vi "Archon RAW to FITS MAIN.vi"() -> ()   [LabVIEW 2023]
uses:
  gfitsio.lvlib
  cfitsio-bitpix.ctl
  gfitsio-write-image-subset-i16-2d.vi
  <vilib>/picture/picture.llb/Draw True-Color Pixmap.vi
  gfitsio-read-image-subset-i32-2d.vi
panel:
  out "hdu names":string[](array[string])=["Primary", "test3.fits"]
  out "hdu name":string="test3.fits"
  in  "Tab Control":enum32{"Complete Image", "Red", "Green", "Blue"}(tab)
  out "Complete Image":picture
  out "Red":picture
  out "Green":picture
  out "Blue":picture
  in  "save binary":path=path "D:/OCI Backups/600__2018_03_12-12.51.07.bin"
  out "Image Data":u16[][](graph)
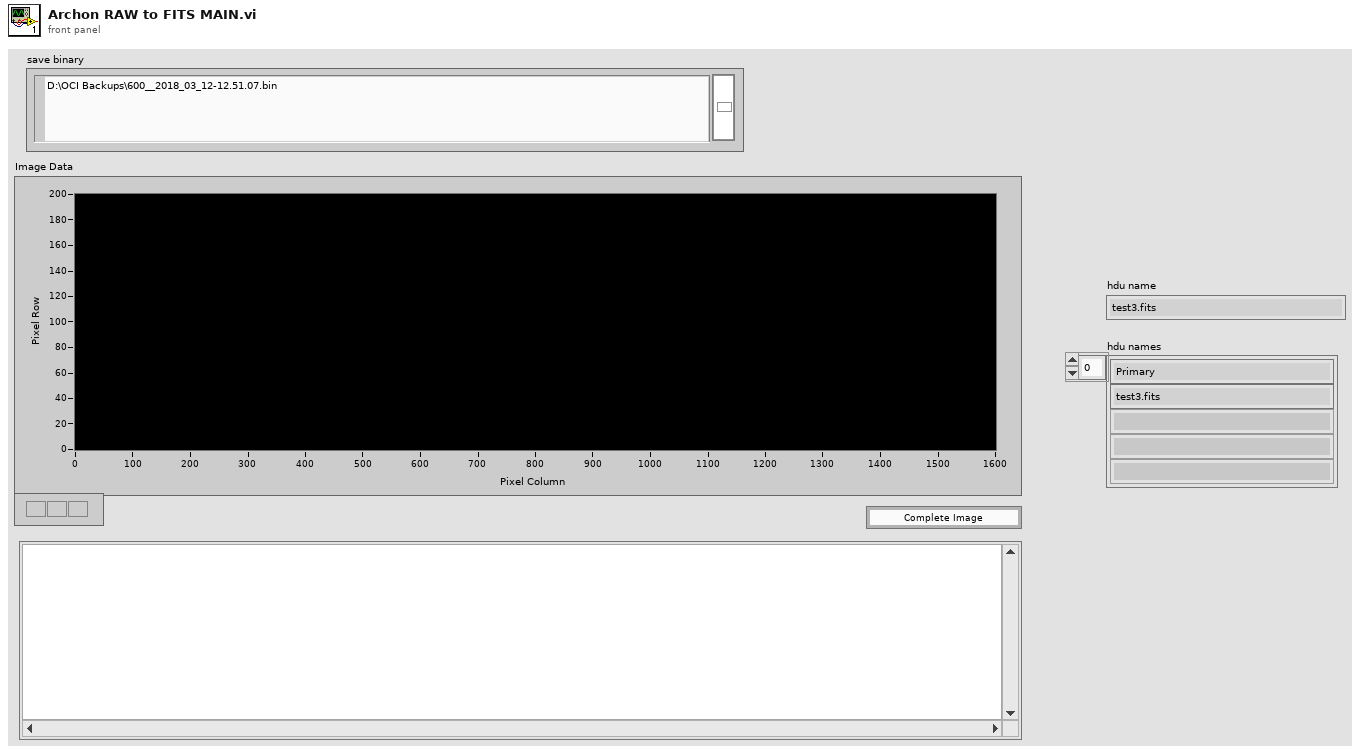
[diagram p1: front panel]
types:
  T1 = enum16{"big-endian, network order", "native, host order", "little-endian"}
  T2 = enum16{"open", "replace", "create", "open or create", "replace or create", "replace or create with confirmation"}
  T3 = enum16{"open", "open or create", "create", "create or replace"}
  T4 = enum16{"open", "open or create", "create or replace", "create", "open (read only)"}
  T5 = typedef "gfitsio.lvlib/cfitsio-bitpix.ctl" = i32
  T6 = typedef "gfitsio.lvlib/gfitsio-refnum.ctl" = refnum<k1>
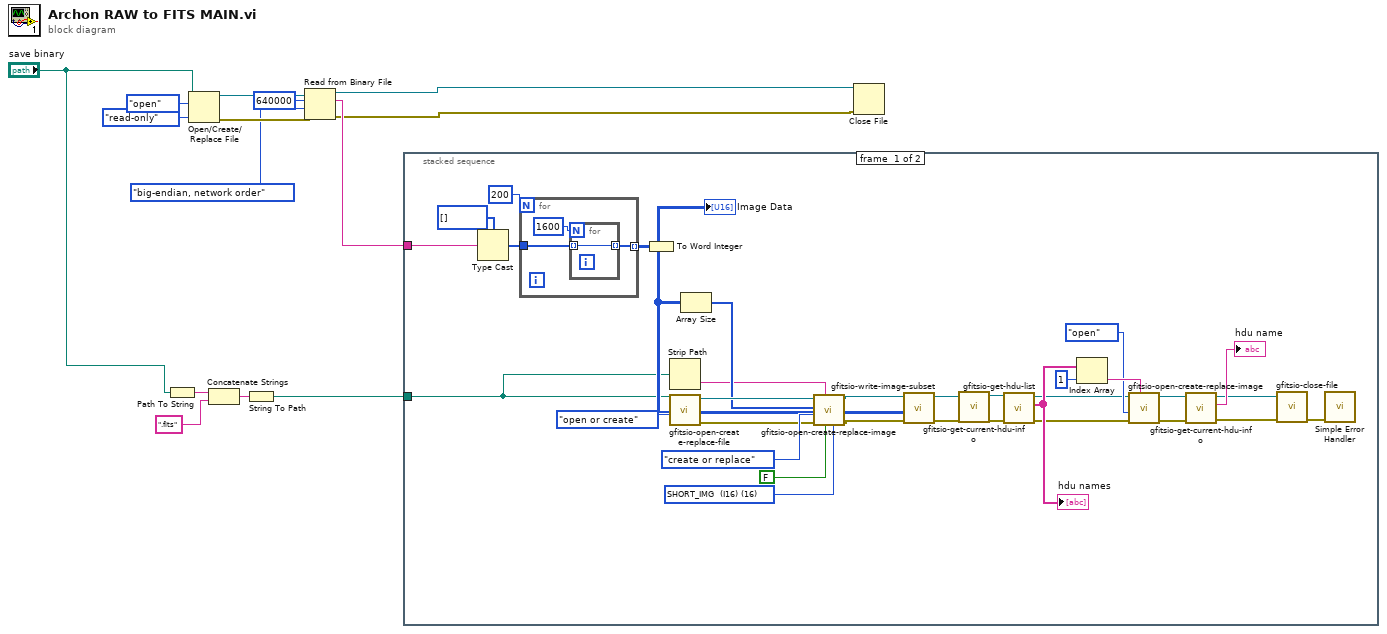
[diagram p0: block diagram]
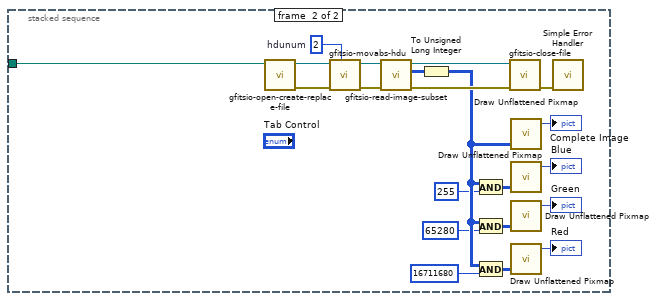
[diagram p2: hidden frame]
diagram:
  n1 = Path To String(path="save binary") -> (string=w5:string)
  n2 = Open/Create/Replace File(file path (use dialog)="save binary", operation (0:open)=T2."open", access (0:read/write)=enum16{"read/write", "read-only", "write-only"}."read-only") -> (refnum out=w12:refnum<file>, error out=w11:errorcluster)  [unwired: 3 in, 1 out]
  n3 = Concatenate Strings(w5, ".fits" ("string")) -> (w3:string)
  n4 = String To Path(string=w3) -> (path=w1:path)
  n5 = Read from Binary File(8:w11, 9:T1."big-endian, network order" ("byte order (0:big-endian, network order)"), 10:640000 ("count (1)"), 11:w12) -> (0:w6:errorcluster, 2:w8:string, 3:w7:refnum<file>)  [unwired: 2 in, 1 out]
  n6 = stacked-sequence {
    tunnel: w8 -> [w45 _]
    tunnel: w1 -> [w15 w51]
    frame #0 {
      w41 = T5 16 items=["<invalid type>"=0, "BYTE_IMG  (U8)"=8, "SHORT_IMG  (I16)"=16, "USHORT_IMG  (U16)"=20, "LONG_IMG  (I32)"=32, "ULONG_IMG  (U32)"=40, "FLOAT_IMG  (SGL)"=-32, "DOUBLE_IMG  (DBL)"=-64] ("image data type")
      n7 = Type Cast(type=u16[] [], x=w45) -> (*(type *) &x=w44:u16[])
      n8 = for {
        N: 200 ("dimension size") -> [_]
        tunnel: w44 -> [w49]
        tunnel: [w48] -> w18 mode=indexing
        n9 = for {
          N: 1600 ("dimension size") -> [_]
          tunnel: w49 -> [w50] mode=indexing
          tunnel: [w50] -> w48 mode=indexing
        }
      }
      "Image Data" <- w18
      n10 = To Word Integer(number=w18) -> ()  [unwired: 1 out]
      n11 = Strip Path(path=w15) -> (name=w16:string)  [unwired: 1 out]
      n12 = call "gfitsio-open-create-replace-file.vi"("function (open)"=T4."open or create", "file path (dialog if empty)"=w15) -> ("error out"=w38:errorcluster, "gfits refnum"=w37:T6)  [unwired: 7 in, 1 out]
      n13 = Array Size(array=w18) -> (size(s)=w36:i32[])
      n14 = call "gfitsio-open-create-replace-image.vi"("image data type"=w41, "advisory dialog? (display:T)"=FALSE, "hdu name (dialog if empty)"=w16, "error in (no error)"=w38, "function (create or replace)"=T3."create or replace" ("function (open or create)"), "naxes"=w36, "gfits refnum"=w37) -> ("error out"=w19:errorcluster, "dup gfits refnum"=w20:T6)  [unwired: 2 in, 1 out]
      n15 = call-poly "gfitsio-write-image-subset.vi"("error in (no error)"=w19, "data"=w18, "gfits refnum"=w20) -> ("error out"=w23:errorcluster, "dup gfits refnum"=w22:T6)  [unwired: 7 in]
      n16 = call "gfitsio-get-current-hdu-info.vi"("error in (no error)"=w23, "gfits refnum"=w22) -> ("error out"=w25:errorcluster, "dup gfits refnum"=w24:T6)  [unwired: 5 in, 3 out]
      n17 = call "gfitsio-get-hdu-list.vi"("error in (no error)"=w25, "gfits refnum"=w24) -> ("error out"=w27:errorcluster, "hdu names"=w33:string[], "dup gfits refnum"=w26:T6)  [unwired: 6 in, 1 out]
      "hdu names" <- w33
      n18 = Index Array(array=w33, index=1) -> (element=w34:string)
      n19 = call "gfitsio-open-create-replace-image.vi"("hdu name (dialog if empty)"=w34, "error in (no error)"=w27, "function (create or replace)"=T3."open", "gfits refnum"=w26) -> ("error out"=w30:errorcluster, "dup gfits refnum"=w29:T6)  [unwired: 5 in, 1 out]
      n20 = call "gfitsio-get-current-hdu-info.vi"("error in (no error)"=w30, "gfits refnum"=w29) -> ("error out"=w31:errorcluster, "hdu name"=→"hdu name":string, "dup gfits refnum"=w17:T6)  [unwired: 5 in, 2 out]
      n21 = call "gfitsio-close-file.vi"("error in (no error)"=w31, "gfits refnum"=w17) -> ("error out"=w21:errorcluster)  [unwired: 8 in, 1 out]
      n22 = call <vilib>:"Simple Error Handler.vi"("error in (no error)"=w21) -> ()  [unwired: 4 in, 5 out]
    }
    frame #1 {
      w52 = 2  # hdunum
      n23 = call "gfitsio-open-create-replace-file.vi"("file path (dialog if empty)"=w51) -> ("error out"=w71:errorcluster, "gfits refnum"=w70:T6)  [unwired: 8 in, 1 out]
      n24 = call "gfitsio-movabs-hdu.vi"("hdunum"=w52, "error in (no error)"=w71, "gfits refnum"=w70) -> ("error out"=w69:errorcluster, "dup gfits refnum"=w68:T6)  [unwired: 6 in, 1 out]
      n25 = call-poly "gfitsio-read-image-subset.vi"("error in (no error)"=w69, "gfits refnum"=w68) -> ("error out"=w67:errorcluster, "data"=w64:i32[][], "dup gfits refnum"=w66:T6)  [unwired: 7 in]
      n26 = To Unsigned Long Integer(number=w64) -> (unsigned 32bit integer=w56:u32[][])
      n27 = And(x=w56, y=u32 255) -> (x .and. y?=w63:u32[][])
      n28 = And(x=w56, y=u32 65280) -> (x .and. y?=w60:u32[][])
      n29 = And(x=w56, y=u32 16711680) -> (x .and. y?=w58:u32[][])
      n30 = call "gfitsio-close-file.vi"("error in (no error)"=w67, "gfits refnum"=w66) -> ("error out"=w65:errorcluster)  [unwired: 8 in, 1 out]
      n31 = call-poly <vilib>:"Draw Unflattened Pixmap.vi"("data (RGB format)"=w56) -> ("new picture"=→"Complete Image":picture)  [unwired: 8 in]
      n32 = call-poly <vilib>:"Draw Unflattened Pixmap.vi"("data (RGB format)"=w63) -> ("new picture"=→"Blue":picture)  [unwired: 8 in]
      n33 = call-poly <vilib>:"Draw Unflattened Pixmap.vi"("data (RGB format)"=w60) -> ("new picture"=→"Green":picture)  [unwired: 8 in]
      n34 = call-poly <vilib>:"Draw Unflattened Pixmap.vi"("data (RGB format)"=w58) -> ("new picture"=→"Red":picture)  [unwired: 8 in]
      n35 = call <vilib>:"Simple Error Handler.vi"("error in (no error)"=w65) -> ()  [unwired: 4 in, 5 out]
    }
  }
  n36 = Close File(refnum=w7, error in=w6) -> ()  [unwired: 2 out]
